vi "Servo check errors.vi"(11 "connection in":variant) -> (0 "error out":errorcluster, 1 "diagnosis text":string, 2 "OK":bool, 3 "connection out":variant)   [LabVIEW 2022 SP3, in "Servo drive module.lvlib"]
doc: "Checks for errors that may occure in physical controller of servo drive. Resolve errors caused by reaching of limits. Other errors are send to output."
uses:
  Servo drive module.lvlib
  <vilib>/addons/eal4LabVIEW/eal4LabVIEW.lvlib
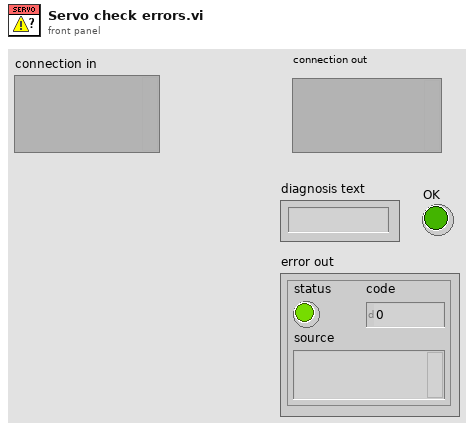
[diagram p1: front panel]
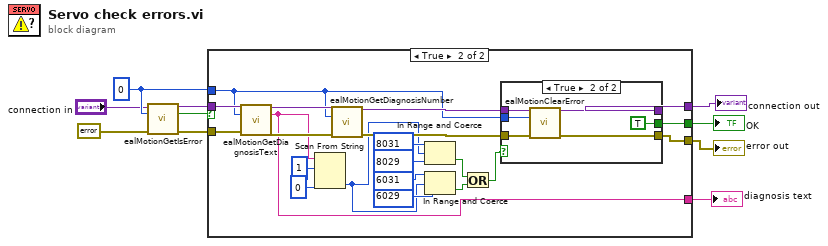
[diagram p0: block diagram]
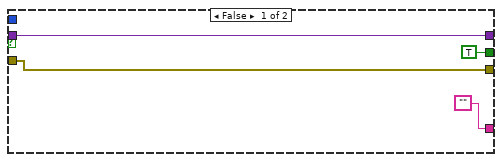
[diagram p2: hidden frame]
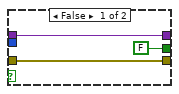
[diagram p3: hidden frame]
diagram:
  w8 = 0 ("slave index")
  n1 = call <vilib>:"ealMotionGetIsError.vi"("connection in"="connection in", "slave index"=w8, "error in (no error)"=errorcluster {"status"=FALSE, "code"=0, "source"=""}) -> ("connection out"=w6:variant, "error"=w5:bool, "error out"=w7:errorcluster)  [unwired: 10 in]
  n2 = case shown="True" w5 {
    tunnel: w6 -> [w14 w35]
    tunnel: w7 -> [w13 w34]
    tunnel: w8 -> [_ w27]
    tunnel: [w14 w33] -> w2
    tunnel: [w13 w32] -> w9
    tunnel: ["" w17] -> w10
    tunnel: [TRUE w24] -> w1
    frame False {
    }
    frame True {
      n3 = call <vilib>:"ealMotionGetDiagnosisText.vi"("connection in"=w35, "slave index"=w27, "error in (no error)"=w34) -> ("connection out"=w30:variant, "diagnosis text"=w17:string, "error out"=w29:errorcluster)  [unwired: 10 in]
      n4 = Scan From String(input string=w17, initial scan location=u32 1, default 1=0) -> (output 1=w16:i32)  [unwired: 2 in, 3 out]
      n5 = call <vilib>:"ealMotionGetDiagnosisNumber.vi"("connection in"=w30, "slave index"=w27, "error in (no error)"=w29) -> ("connection out"=w31:variant, "error out"=w28:errorcluster)  [unwired: 10 in, 1 out]
      n6 = In Range and Coerce(upper limit=8031, x=w16, lower limit=8029) -> (In Range?=w23:bool)  [unwired: 1 out]
      n7 = In Range and Coerce(upper limit=6031 ("y"), x=w16, lower limit=6029 ("y")) -> (In Range?=w20:bool)  [unwired: 1 out]
      n8 = Or(x=w23, y=w20) -> (x .or. y?=w15:bool)
      n9 = case shown="True" w15 {
        tunnel: [w38 w44] -> w33
        tunnel: [w37 w43] -> w32
        tunnel: w31 -> [w38 w42]
        tunnel: w28 -> [w37 w41]
        tunnel: w27 -> [_ w40]
        tunnel: [FALSE TRUE] -> w24
        frame False {
        }
        frame True {
          n10 = call <vilib>:"ealMotionClearError.vi"("connection in"=w42, "slave index"=w40, "error in (no error)"=w41) -> ("connection out"=w44:variant, "error out"=w43:errorcluster)  [unwired: 11 in]
        }
      }
    }
  }
  "diagnosis text" <- w10
  "error out" <- w9
  "connection out" <- w2
  "OK" <- w1
